vi "Init.vi"(8 "error in":errorcluster, 11 "Virtual Thermometer from CSV in":refnum<class "Virtual Sensor from CSV.lvclass">) -> (0 "error out":errorcluster, 3 "Virtual Thermometer from CSV out":refnum<class "Virtual Sensor from CSV.lvclass">)   [LabVIEW 2024, in "Virtual Sensor from CSV.lvclass"]
uses:
  Virtual Sensor from CSV.lvclass
  Virtual Sensor from CSV.lvclass/Virtual Sensor from CSV.ctl
  Interfaces/IConfiguration/IConfiguration.lvclass
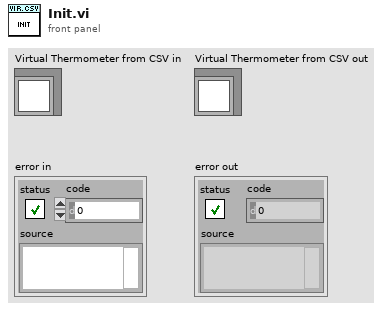
[diagram p1: front panel]
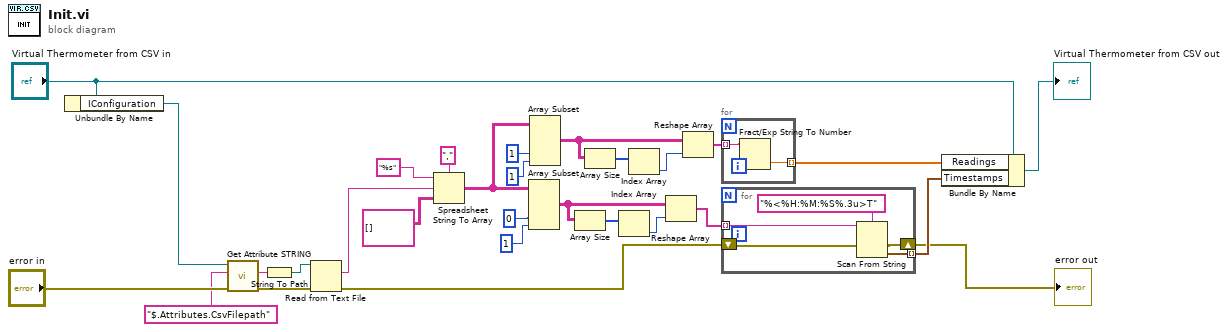
[diagram p0: block diagram]
diagram:
  n1 = Unbundle By Name("Virtual Thermometer from CSV in") -> ("IConfiguration"=w1:refnum<class "IConfiguration.lvclass">)
  n2 = call-dynamic "Get Attribute STRING.vi"("error in"="error in", "Attribute"="$.Attributes.CsvFilepath", "IConfiguration in"=w1) -> ("error out"=w27:errorcluster, "Value"=w26:string)  [unwired: 6 in, 1 out]
  n3 = String To Path(string=w26) -> (path=w22:path)
  n4 = Read from Text File(file (use dialog)=w22, error in=w27) -> (text=w21:string, error out=w4:errorcluster)  [unwired: 2 in, 2 out]
  n5 = Spreadsheet String To Array(delimiter (Tab)=",", format string="%s", spreadsheet string=w21, array type (2D Dbl)=string[][] []) -> (array=w18:string[][])
  n6 = Array Subset(array=w18, index (col)=0 ("index"), length (col)=1 ("length")) -> (w8:string[][])  [unwired: 2 in]
  n7 = Array Subset(array=w18, index (col)=1 ("index"), length (col)=1 ("length")) -> (w15:string[][])  [unwired: 2 in]
  n8 = Array Size(array=w8) -> (size(s)=w9:i32[])
  n9 = Array Size(array=w15) -> (size(s)=w14:i32[])
  n10 = Index Array(array=w9) -> (element=w7:i32)  [unwired: 1 in]
  n11 = Index Array(array=w14) -> (element=w13:i32)  [unwired: 1 in]
  n12 = Reshape Array(w8, w7) -> (w6:string[])
  n13 = Reshape Array(w15, w13) -> (w12:string[])
  n14 = for {
    tunnel: w12 -> [w31] mode=indexing
    tunnel: [w30] -> w10 mode=indexing
    n15 = Fract/Exp String To Number(string=w31) -> (number=w30:dbl)  [unwired: 3 in, 1 out]
  }
  n16 = for {
    tunnel: w6 -> [w36] mode=indexing
    tunnel: [w35] -> w5 mode=indexing
    shift-right: [w33] -> w3
    shift-left: w4 -> [w34]
    n17 = Scan From String(format string="%<%H:%M:%S%.3u>T", input string=w36, error in=w34) -> (error out=w33:errorcluster, output 1=w35:timestamp)  [unwired: 2 in, 2 out]
  }
  "error out" <- w3
  n18 = Bundle By Name(cluster="Virtual Thermometer from CSV in", "Readings"=w10, "Timestamps"=w5) -> (→"Virtual Thermometer from CSV out":refnum<class "Virtual Sensor from CSV.lvclass">)
